vi "Generate Waveform.vi"(0 "signal configuration":refnum<class "SV Triangle.lvclass">, 5 "template waveform":waveform(dbl), 9 "samples":i32, 11 "error in (no error)":errorcluster) -> (4 "signal configuration":refnum<class "SV Triangle.lvclass">, 6 "triangle waveform":waveform(dbl), 10 "samples":i32, 15 "error out":errorcluster)   [LabVIEW 2017, in "SV Triangle.lvclass"]
uses:
  <vilib>/addons/_NISVFA/_Generation/Signal Generation/SV Triangle/SV Triangle.lvclass
  C:/Program Files (x86)/National Instruments/LabVIEW 2017/vi.lib/addons/_NISVFA/_Generation/Signal Generation/SV Signal/SV Signal.lvclass
  C:/Program Files (x86)/National Instruments/LabVIEW 2017/vi.lib/addons/_NISVFA/_Generation/Signal Generation/SV Function/SV Function.lvclass
  <vilib>/addons/_NISVFA/_Generation/Signal Generation/SV Signal/sv_Signal State Attribute.ctl
  <vilib>/addons/_NISVFA/_Generation/Signal Generation/SV Triangle/SV Triangle.lvclass/SV Triangle.ctl
  <vilib>/addons/_NISVFA/_Generation/Signal Generation/SV Signal/Read Sample Rate.vi
  <vilib>/addons/_NISVFA/_Generation/Signal Generation/SV Function/SV Function.lvclass
  <vilib>/addons/_NISVFA/_Generation/Signal Generation/SV Signal/SV Signal.lvclass
  <vilib>/Analysis/NI_AALBase.lvlib
  <vilib>/measure/NI_MABase.lvlib
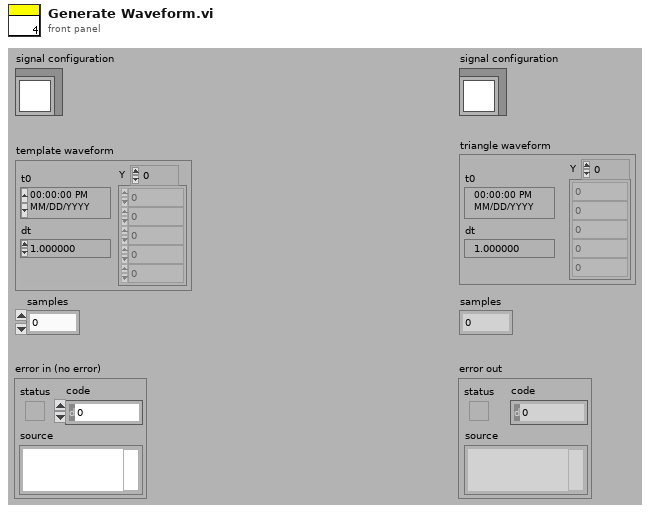
[diagram p1: front panel]
types:
  T1 = typedef "SV Signal.lvclass/sv_Signal State Attribute.ctl" = string
  T2 = typedef "SV Signal.lvclass/sv_System Timing Model.ctl" = i64
  T3 = typedef "SV Signal.lvclass/sv_Generation State.ctl" = enum16{"Idle", "Ramp Up", "Pre-Measurement Settling", "Measurement", "Post-Measurement Settling", "Discrete Sweep Transition", "Ramp Down", "Update"}
  T4 = cluster{"system timing model":T2, "state":cluster{"RESET":bool, "generator timestamp":timestamp, "elapsed seconds":dbl, "elapsed samples":u64, "generation state":T3, "time offset at state":dbl, "samples generated at state":u64, "signal state":variant}, "duration of state":dbl, "samples remaining at state":i32}
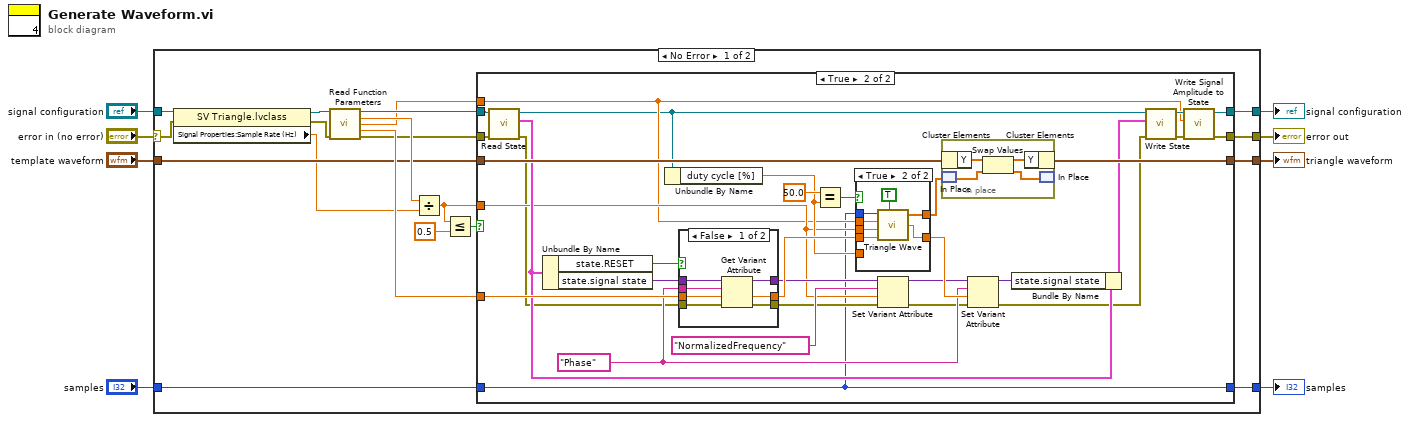
[diagram p0: block diagram]
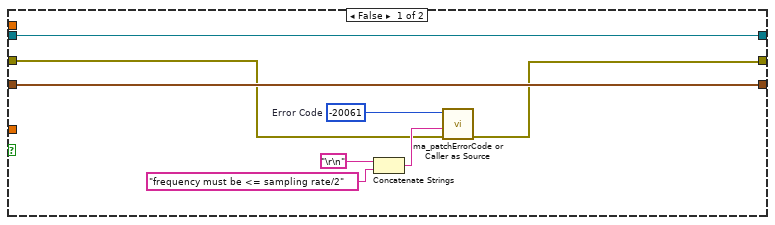
[diagram p2: hidden frame]
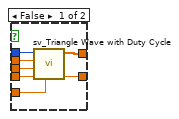
[diagram p3: hidden frame]
diagram:
  n1 = case shown="No Error" "error in (no error)" {
    selector: "error in (no error)" -> [w9 w97]
    tunnel: [w18 w97] -> w3
    tunnel: [w19 w96] -> w7
    tunnel: "signal configuration" -> [w15 w96]
    tunnel: [w27 _] -> w2
    tunnel: [w10 _] -> w1
    tunnel: "samples" -> [w25 _]
    tunnel: "template waveform" -> [w23 _]
    frame No Error {
      n2 = property class="SV Triangle.lvclass"(reference=w15, error in=w9) -> (reference out=w22:refnum<class "SV Triangle.lvclass">, error out=w21:errorcluster, "Signal Properties:Sample Rate (Hz)"=w20:dbl)
      n3 = call <vilib>:"Read Function Parameters.vi"("signal configuration"=w22, "error in (no error)"=w21) -> ("signal configuration"=w14:refnum<class "SV Triangle.lvclass">, "frequency_Hz"=w26:dbl, "amplitude"=w12:dbl, "initial_phase_deg"=w24:dbl, "error out"=w13:errorcluster)  [unwired: 8 in, 1 out]
      n4 = Divide(x=w26, y=w20) -> (x/y=w16:dbl)
      n5 = Less Or Equal?(x=w16, y=0.5) -> (x <= y?=w11:bool)
      n6 = case shown="True" w11 {
        tunnel: [w34 w66] -> w27
        tunnel: w25 -> [_ w41]
        tunnel: w24 -> [_ w64]
        tunnel: w23 -> [w34 w62]
        tunnel: [w35 w40] -> w19
        tunnel: [w28 w39] -> w18
        tunnel: w16 -> [_ w46]
        tunnel: w14 -> [w35 w45]
        tunnel: w13 -> [w29 w44]
        tunnel: w12 -> [_ w42]
        tunnel: [_ w41] -> w10
        frame False {
          w30 = -20061  # Error Code
          n7 = Concatenate Strings("\r\n", "frequency must be <= sampling rate/2" ("freq error message")) -> (w33:string)
          n8 = call <vilib>:"ma_patchErrorCode or Caller as Source.vi"("error in (no error)"=w29, "string to append to source"=w33, "error code"=w30) -> ("error out"=w28:errorcluster)  [unwired: 8 in]
        }
        frame True {
          w58 = T1 "Phase" ("name")
          n9 = call <vilib>:"Read State.vi"("error in (no error)"=w44, "signal configuration"=w45) -> ("error out"=w43:errorcluster, "generator state"=w61:T4, "signal configuration"=w38:refnum<class "SV Triangle.lvclass">)  [unwired: 7 in]
          n10 = Unbundle By Name(w61) -> ("state.RESET"=w36:bool, "state.signal state"=w65:variant)
          n11 = Unbundle By Name(w38) -> ("duty cycle [%]"=w50:dbl)
          n12 = case shown="False" w36 {
            tunnel: w65 -> [w88 w90]
            tunnel: w64 -> [w87 w91]
            tunnel: [w86 w91] -> w63
            tunnel: [w85 w90] -> w57
            tunnel: w43 -> [w84 w89]
            tunnel: [w83 w89] -> w54
            tunnel: w58 -> [w82 _]
            frame False {
              n13 = Get Variant Attribute(Variant=w88, name=w82, default value (empty Variant)=w87, error in=w84) -> (duplicate Variant=w85:variant, value=w86:dbl, error out=w83:errorcluster)  [unwired: 1 out]
            }
            frame True {
            }
          }
          n14 = Equal?(x=50.0 ("y"), y=w50) -> (x = y?=w51:bool)
          n15 = case shown="True" w51 {
            tunnel: [w70 w81] -> w67
            tunnel: w42 -> [w73 w79]
            tunnel: w41 -> [w74 w78]
            tunnel: w63 -> [w71 w77]
            tunnel: [w69 w76] -> w59
            tunnel: w46 -> [w72 w75]
            tunnel: w50 -> [w68 _]
            frame False {
              n16 = call <vilib>:"sv_Triangle Wave with Duty Cycle.vi"("duty cycle [%]"=w68, "phase in [deg]"=w71, "normalized frequency (f/Fs)"=w72, "amplitude"=w73, "samples"=w74) -> ("phase out"=w69:dbl, "triangle wave"=w70:dbl[])  [unwired: 5 in]
            }
            frame True {
              n17 = call <vilib>:"Triangle Wave.vi"("samples"=w78, "amplitude"=w79, "frequency"=w75, "phase in"=w77, "reset phase"=TRUE) -> ("triangle wave"=w81:dbl[], "phase out"=w76:dbl)  [unwired: 1 out]
            }
          }
          n18 = Set Variant Attribute(Variant=w57, name=T1 "NormalizedFrequency", value=w46, error in=w54) -> (Variant out=w56:variant, error out=w53:errorcluster)  [unwired: 1 out]
          n19 = in-place {
            n20 = in-place-cluster #1(w62) -> ("Y"=w95:dbl[])
            n21 = in-place-match #2(w67) -> (w93:dbl[])
            n22 = Swap Values(12:w95, 14:w93) -> (1:w94:dbl[], 3:w92:dbl[])  [unwired: 1 in]
            n23 = in-place-cluster #1("Y"=w94) -> (w66:waveform(dbl))
            n24 = in-place-match #2(w92) -> ()  [unwired: 1 out]
          }
          n25 = Set Variant Attribute(Variant=w56, name=w58, value=w59, error in=w53) -> (Variant out=w60:variant, error out=w37:errorcluster)  [unwired: 1 out]
          n26 = Bundle By Name(cluster=w61, "state.signal state"=w60) -> (w49:T4)
          n27 = call <vilib>:"Write State.vi"("error in (no error)"=w37, "generator state"=w49, "signal configuration"=w38) -> ("error out"=w47:errorcluster, "signal configuration"=w48:refnum<class "SV Triangle.lvclass">)  [unwired: 7 in]
          n28 = call <vilib>:"Write Signal Amplitude to State.vi"("error in (no error)"=w47, "amplitude"=w42, "SV Signal in"=w48) -> ("error out"=w39:errorcluster, "SV Signal out"=w40:refnum<class "SV Triangle.lvclass">)  [unwired: 7 in]
        }
      }
    }
    frame Error {
    }
  }
  "error out" <- w3
  "signal configuration" <- w7
  "triangle waveform" <- w2
  "samples" <- w1
